vi "Maszyna stanu.vi"() -> ()   [LabVIEW 2020]
uses:
  Controlka.ctl
panel:
  in  "stop":bool
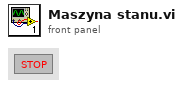
[diagram p1: front panel]
types:
  T1 = typedef "Controlka.ctl" = enum16{""}
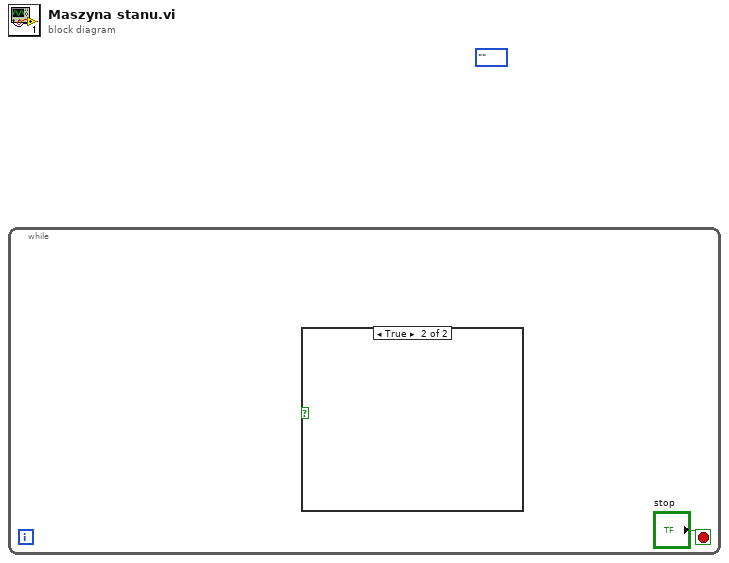
[diagram p0: block diagram]
diagram:
  (unwired) Controlka.""
  n1 = while {
    stop <- "stop" stop-if-true
    n2 = case shown="True" {
      selector: _ -> [_ _]
      frame False {
      }
      frame True {
      }
    }
  }
